vi "Set Footer Object Positions.vi"(4 "FP.width":i16, 8 "error in":errorcluster, 9 "SR List.height":u32, 10 "label array in":string[](array[string]), 11 "controls[] in":refnum<vi>[](array[refnum])) -> (0 "error out":errorcluster)   [LabVIEW 2018]
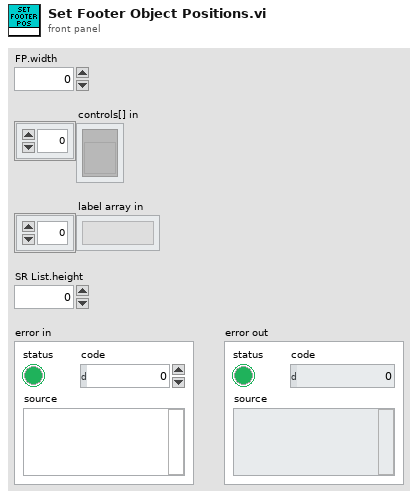
[diagram p1: front panel]
types:
  T1 = typedef "LVRectTypeDef.ctl" = cluster{"Left":i16, "Top":i16, "Right":i16, "Bottom":i16}
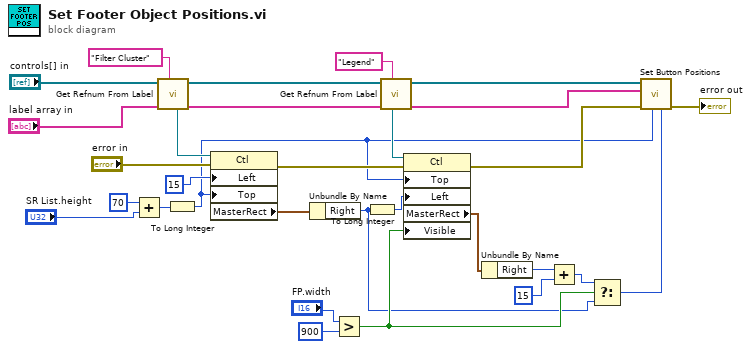
[diagram p0: block diagram]
diagram:
  n1 = Add(x=u32 70, y="SR List.height") -> (x+y=w7:u32)
  n2 = call "Get Refnum From Label.vi"("label"="Filter Cluster" ("element"), "label array in"="label array in", "controls[] in"="controls[] in") -> ("label array out"=w12:string[], "controls[] out"=w10:refnum<vi>[], "refnum out"=w23:refnum<vi>)  [unwired: 6 in]
  n3 = To Long Integer(number=w7) -> (32bit integer=w1:i32)
  n4 = property class="Ctl"(reference=w23, error in="error in", "Left"=15 ("Position:Left"), "Top"=w1) -> (error out=w4:errorcluster, "MasterRect"=w9:T1)  [unwired: 1 out]
  n5 = Unbundle By Name(w9) -> ("Right"=w21:i16)
  n6 = Greater?(x="FP.width", y=i16 900) -> (0:w25:bool)
  n7 = To Long Integer(number=w21) -> (32bit integer=w16:i32)
  n8 = call "Get Refnum From Label.vi"("label"="Legend", "label array in"=w12, "controls[] in"=w10) -> ("label array out"=w13:string[], "controls[] out"=w14:refnum<vi>[], "refnum out"=w11:refnum<vi>)  [unwired: 6 in]
  n9 = property class="Ctl"(reference=w11, error in=w4, "Top"=w1, "Left"=w16, "Visible"=w25) -> (error out=w3:errorcluster, "MasterRect"=w17:T1)  [unwired: 1 out]
  n10 = Unbundle By Name(w17) -> ("Right"=w18:i16)
  n11 = Add(x=w18, y=i16 15) -> (x+y=w20:i16)
  n12 = Select(t=w20, s=w25, f=w21) -> (s? t:f=w2:i16)
  n13 = call "Set Button Positions.vi"("Left"=w2, "Top"=w1, "error in"=w3, "label array in"=w13, "controls[] in"=w14) -> ("error out"=→"error out":errorcluster)  [unwired: 6 in]
